vi "LinearSVC.vi"(8 "error in":errorcluster) -> (0 "error out":errorcluster, 3 "out":refnum<class "LinearSVC.lvclass">)   [LabVIEW 2020]
doc: "Linear Support Vector Classification.\n\n Similar to SVC with parameter kernel='linear', but implemented in terms of\n liblinear rather than libsvm, so it has more flexibility in the choice of\n penalties and loss functions and should scale better to large numbers of\n samples.\n\n This class supports both dense and sparse input and the multiclass support\n is handled according to a one-vs-the-rest scheme.\n\n Read more in the :ref:`User Guide <svm_classification>`.\n\n Parameters\n ----------\n penalty : {'l1', 'l2'}, default='l2'\n Specifies the norm used in the penalization. The 'l2'\n penalty is the standard used in SVC. The 'l1' leads to ``coef_``\n vectors that are sparse.\n\n loss : {'hinge', 'squared_hinge'}, default='squared_hinge'\n Specifies the loss function. 'hinge' is the standard SVM loss\n (used e.g. by the SVC class) while 'squared_hinge' is the\n square of the hinge loss. The combination of ``penalty='l1'``\n and ``loss='hinge'`` is not supported.\n\n dual : bool, default=True\n Select the algorithm to either solve the dual or primal\n optimization problem. Prefer dual=False when n_samples > n_features.\n\n tol : float, default=1e-4\n Tolerance for stopping criteria.\n\n C : float, default=1.0\n Regularization parameter. The strength of the regularization is\n inversely proportional to C. Must be strictly positive.\n\n multi_class : {'ovr', 'crammer_singer'}, default='ovr'\n Determines the multi-class strategy if `y` contains more than\n two classes.\n ``\"ovr\"`` trains n_classes one-vs-rest classifiers, while\n ``\"crammer_singer\"`` optimizes a joint objective over all classes.\n While `crammer_singer` is interesting from a theoretical perspective\n as it is consistent, it is seldom used in practice as it rarely leads\n to better accuracy and is more expensive to compute.\n If ``\"crammer_singer\"`` is chosen, the options loss, penalty and dual\n will be ignored.\n\n fit_intercept : bool, default=True\n Whether to calculate the intercept for this model. If set\n to false, no intercept will be used in calculations\n (i.e. data is expected to be already centered).\n\n intercept_scaling : float, default=1\n When self.fit_intercept is True, instance vector x becomes\n ``[x, self.intercept_scaling]``,\n i.e. a \"synthetic\" feature with constant value equals to\n intercept_scaling is appended to the instance vector.\n The intercept becomes intercept_scaling * synthetic feature weight\n Note! the synthetic feature weight is subject to l1/l2 regularization\n as all other features.\n To lessen the effect of regularization on synthetic feature weight\n (and therefore on the intercept) intercept_scaling has to be increased.\n\n class_weight : dict or 'balanced', default=None\n Set the parameter C of class i to ``class_weight[i]*C`` for\n SVC. If not given, all classes are supposed to have\n weight one.\n The \"balanced\" mode uses the values of y to automatically adjust\n weights inversely proportional to class frequencies in the input data\n as ``n_samples / (n_classes * np.bincount(y))``.\n\n verbose : int, default=0\n Enable verbose output. Note that this setting takes advantage of a\n per-process runtime setting in liblinear that, if enabled, may not work\n properly in a multithreaded context.\n\n random_state : int, RandomState instance or None, default=None\n Controls the pseudo random number generation for shuffling the data for\n the dual coordinate descent (if ``dual=True``). When ``dual=False`` the\n underlying implementation of :class:`LinearSVC` is not random and\n ``random_state`` has no effect on the results.\n Pass an int for reproducible output across multiple function calls.\n See :term:`Glossary <random_state>`.\n\n max_iter : int, default=1000\n The maximum number of iterations to be run.\n\n Attributes\n ----------\n coef_ : ndarray of shape (1, n_features) if n_classes == 2 else (n_classes, n_features)\n Weights assigned to the features (coefficients in the primal\n problem).\n\n ``coef_`` is a readonly property derived from ``raw_coef_`` that\n follows the internal memory layout of liblinear.\n\n intercept_ : ndarray of shape (1,) if n_classes == 2 else (n_classes,)\n Constants in decision function.\n\n classes_ : ndarray of shape (n_classes,)\n The unique classes labels.\n\n n_iter_ : int\n Maximum number of iterations run across all classes.\n\n See Also\n --------\n SVC : Implementation of Support Vector Machine classifier using libsvm:\n the kernel can be non-linear but its SMO algorithm does not\n scale to large number of samples as LinearSVC does.\n\n Furthermore SVC multi-class mode is implemented using one\n vs one scheme while LinearSVC uses one vs the rest. It is\n possible to implement one vs the rest with SVC by using the\n :class:`~sklearn.multiclass.OneVsRestClassifier` wrapper.\n\n Finally SVC can fit dense data without memory copy if the input\n is C-contiguous. Sparse data will still incur memory copy though.\n\n sklearn.linear_model.SGDClassifier : SGDClassifier can optimize the same\n cost function as LinearSVC\n by adjusting the penalty and loss parameters. In addition it requires\n less memory, allows incremental (online) learning, and implements\n various loss functions and regularization regimes.\n\n Notes\n -----\n The underlying C implementation uses a random number generator to\n select features when fitting the model. It is thus not uncommon\n to have slightly different results for the same input data. If\n that happens, try with a smaller ``tol`` parameter.\n\n The underlying implementation, liblinear, uses a sparse internal\n representation for the data that will incur a memory copy.\n\n Predict output may not match that of standalone liblinear in certain\n cases. See :ref:`differences from liblinear <liblinear_differences>`\n in the narrative documentation.\n\n References\n ----------\n `LIBLINEAR: A Library for Large Linear Classification\n <https://www.csie.ntu.edu.tw/~cjlin/liblinear/>`__\n\n \nAvailable methods:\nFit\nPredict\nScore\nGet Attributes\nGet Params\nSet Params"
uses:
  LinearSVC.lvclass
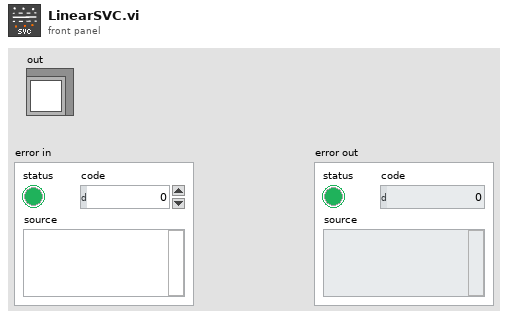
[diagram p1: front panel]
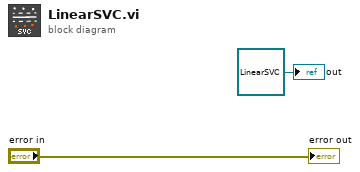
[diagram p0: block diagram]
diagram:
  "out" <- refnum<class "LinearSVC.lvclass"> refnum ("model")
  "error out" <- "error in"
